vi "Generate Multi Commit String.vi"(8 "error in (no error)":errorcluster, 11 "RelayInterface in":refnum<class "RelayInterface.lvclass">[](array[class])) -> (0 "error out":errorcluster)   [LabVIEW 2015, in "RelayInterface.lvclass"]
uses:
  RelayInterface.lvclass
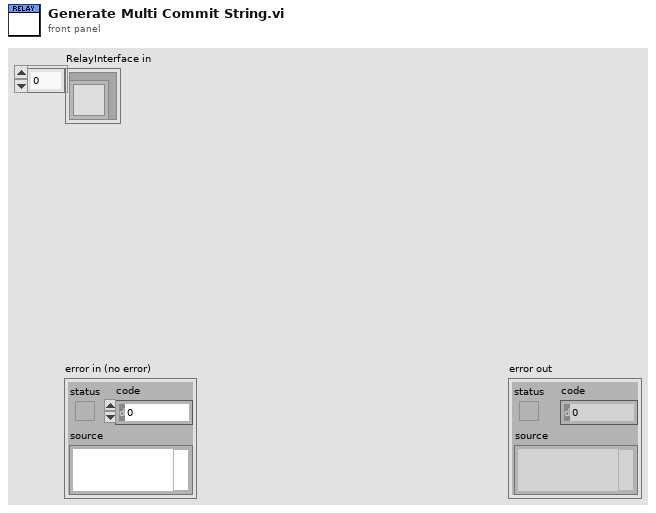
[diagram p1: front panel]
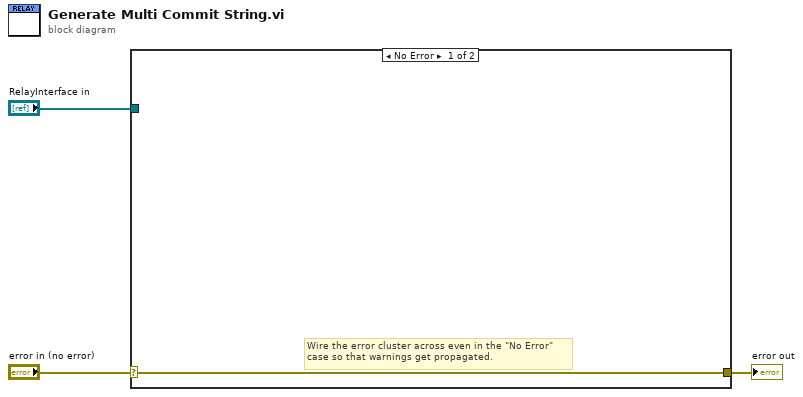
[diagram p0: block diagram]
diagram:
  n1 = case shown="No Error" "error in (no error)" {
    selector: "error in (no error)" -> [w4 w6]
    tunnel: [w4 w6] -> w2
    tunnel: "RelayInterface in" -> [_ w5]
    frame No Error {
      # "Wire the error cluster across even in the \"No Error\"\ncase so that warnings get propagated."
    }
    frame Error {
    }
  }
  "error out" <- w2
